vi "Compile Engine Status.vi"(8 "error in (no error)":errorcluster, 11 "Device Item Ref in":T2 format="%.0x") -> (0 "error out":errorcluster, 2 "Status":T1, 3 "Device Item Ref out":T2 format="%.0x")   [LabVIEW 2019, in "Engine Simulation Toolkit System Explorer.lvlib"]
uses:
  Engine Simulation Toolkit System Explorer.lvlib
  <vilib>/NI VeriStand/Custom Device API/Custom Device Item Ref.ctl
  Shared/Engine Status Data.ctl
  Shared/Constants and GUIDs.vi
  Shared/Engine Simulation Toolkit Shared.lvlib
  <vilib>/NI VeriStand/Custom Device API/Custom Device API.lvlib
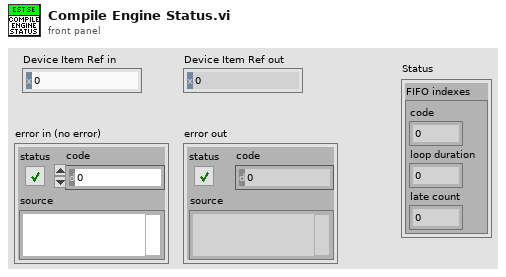
[diagram p1: front panel]
types:
  T1 = typedef "Engine Simulation Toolkit Shared.lvlib/Engine Status Data.ctl" = cluster{"FIFO indexes":cluster{"code":i32, "loop duration":i32, "late count":i32}}
  T2 = typedef "Custom Device API.lvlib/Custom Device Item Ref.ctl" = u64
  T3 = typedef "Engine Simulation Toolkit Shared.lvlib/Channel.ctl" = cluster{"Name":string, "Units":string, "Default":dbl, "Description":string, "Scalable":bool}
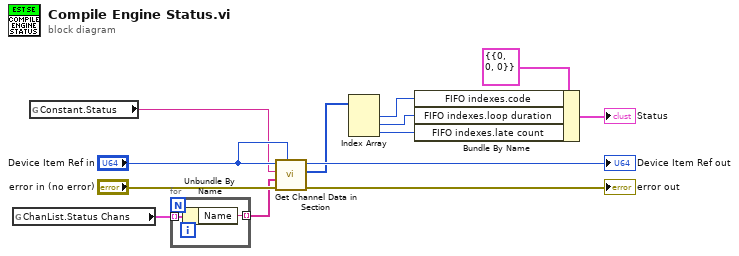
[diagram p0: block diagram]
diagram:
  n1 = global read "Constants and GUIDs.vi" "ChanList.Status Chans"() -> (w6:T3[])
  n2 = global read "Constants and GUIDs.vi" "Constant.Status"() -> (w7:string)
  n3 = for {
    tunnel: w6 -> [w15] mode=indexing
    tunnel: [w14] -> w5 mode=indexing
    n4 = Unbundle By Name(w15) -> ("Name"=w14:string)
  }
  n5 = call "Get Channel Data in Section.vi"("Custom device ref"="Device Item Ref in", "error in (no error)"="error in (no error)", "Channels"=w5, "Section (\"\":none)"=w7, "Item Ref in"="Device Item Ref in") -> ("error out"=→"error out":errorcluster, "FIFO indexes"=w4:i32[], "Item Ref out"=→"Device Item Ref out":T2)  [unwired: 2 in, 2 out]
  n6 = Index Array(array=w4) -> (element #1=w3:i32, element #2=w2:i32, element #3=w1:i32)  [unwired: 3 in]
  n7 = Bundle By Name(cluster=T1 {"FIFO indexes"={"code"=0, "loop duration"=0, "late count"=0}} ("Status"), "FIFO indexes.code"=w3, "FIFO indexes.loop duration"=w2, "FIFO indexes.late count"=w1) -> (→"Status":T1)
